vi "Get Display ROI.vi"() -> ()   [LabVIEW 2020]
uses:
  <vilib>/vision/Image Controls.llb/IMAQ Image.ctl
  Documents/Microscope-Control/Display Module/Display Module Custom Controls/ROI Descriptor.ctl
panel:
  out "Y Center":dbl
  out "X Center":dbl
  out "Height":dbl
  out "Width":dbl
  in  "Quit":bool
  out "Error":bool
  in  "Active Image":u16(ring) items=["Channel 101", "Channel 201"]
  out "ROI Data":i32[](array[numeric])
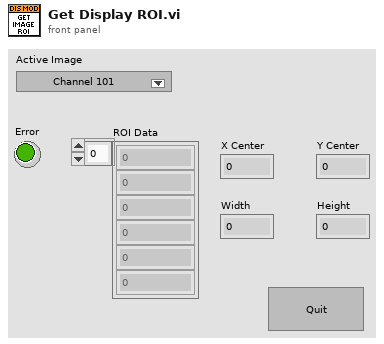
[diagram p1: front panel]
types:
  T1 = typedef "IMAQ Image.ctl" = refnum<image>
  T2 = typedef "ROI Descriptor.ctl" = cluster{"Global Rectangle":i32[], "Contours":cluster{"Contour Type":u32, "ROI Type":u32, "Points":i32[]}[]}
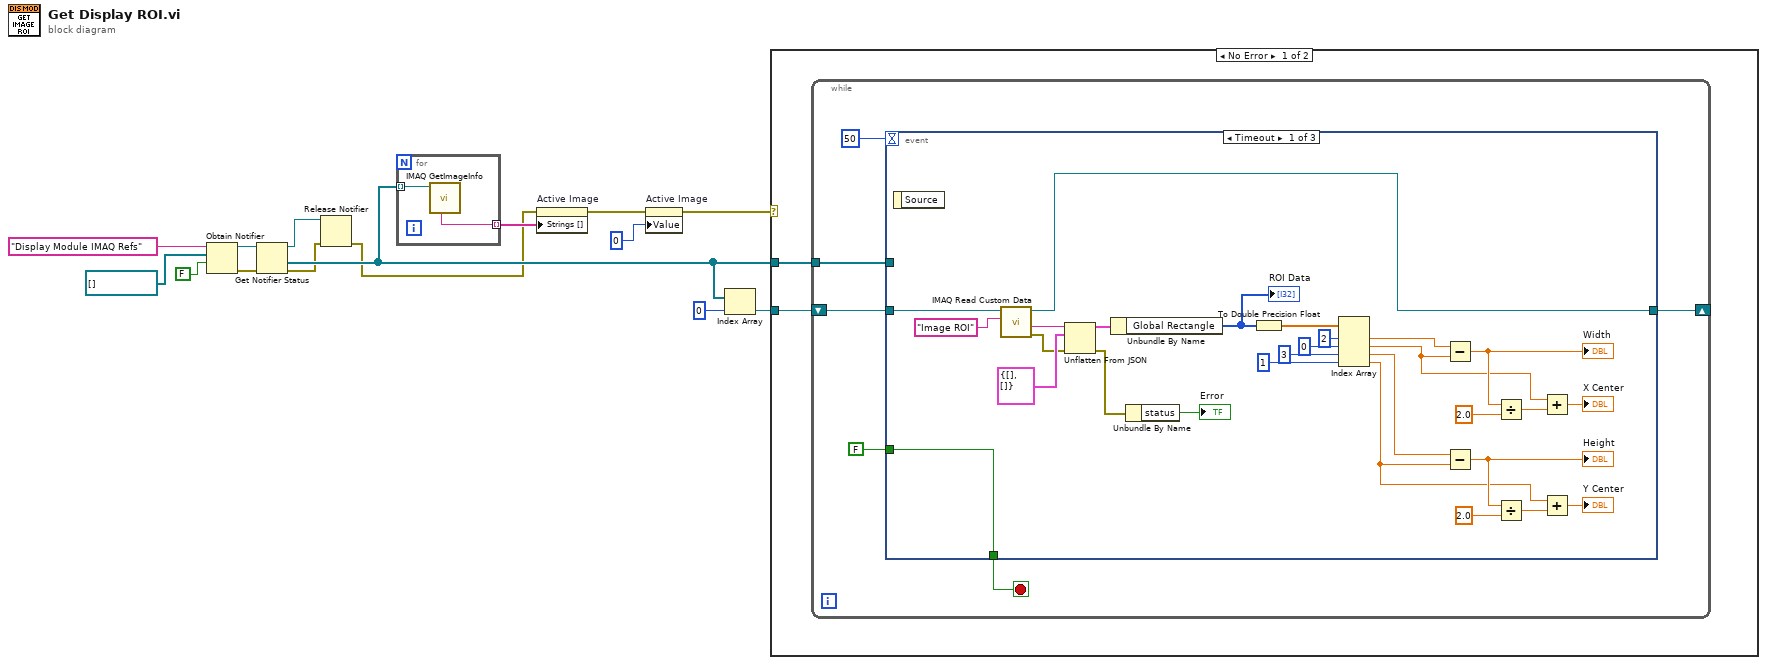
[diagram p0: block diagram]
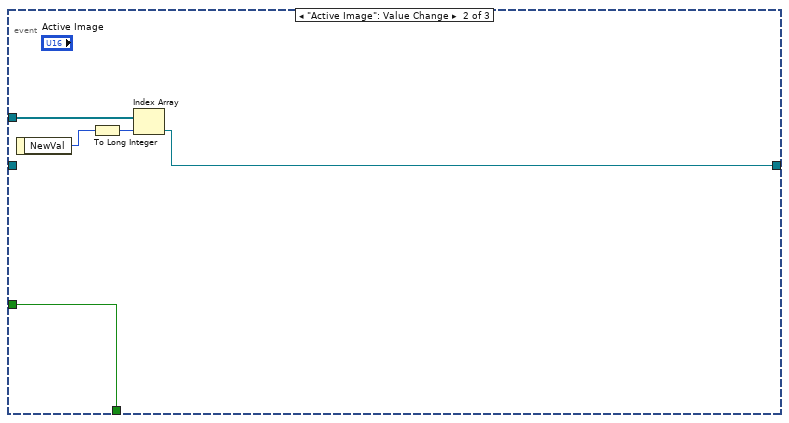
[diagram p2: hidden frame]
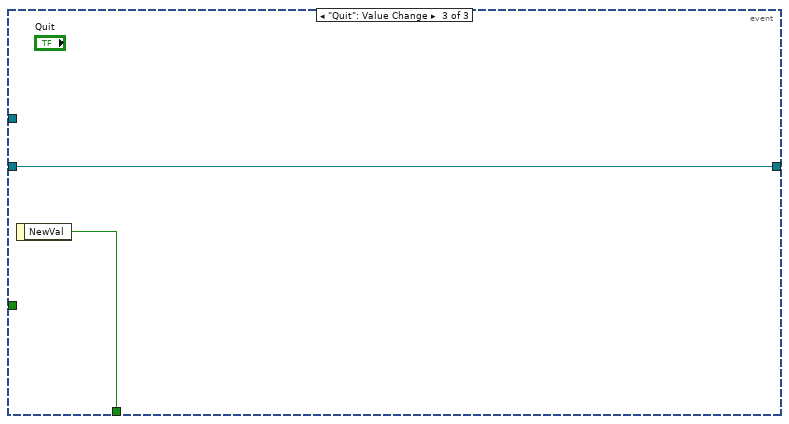
[diagram p3: hidden frame]
diagram:
  n1 = Obtain Notifier(name (unnamed)="Display Module IMAQ Refs", notification data type=T1[] [], create if not found? (T)=FALSE) -> (notifier out=w15:refnum<notifier>, error out=w14:errorcluster)  [unwired: 1 in, 1 out]
  n2 = Get Notifier Status(notifier=w15, error in (no error)=w14) -> (notifier out=w3:refnum<notifier>, current notification=w8:T1[], error out=w2:errorcluster)  [unwired: 2 out]
  n3 = Release Notifier(notifier=w3, error in (no error)=w2) -> (error out=w1:errorcluster)  [unwired: 1 in, 2 out]
  n4 = for {
    tunnel: w8 -> [w17] mode=indexing
    tunnel: [w16] -> w7 mode=indexing
    n5 = call "IMAQ GetImageInfo"("Image"=w17) -> ("Image Name"=w16:string)  [unwired: 3 in, 7 out]
  }
  n6 = property on="Active Image" class="Ring (strict)"(error in=w1, "Strings []"=w7) -> (error out=w5:errorcluster)  [unwired: 1 in, 1 out]
  n7 = property on="Active Image" class="Ring (strict)"(error in=w5, "Value"=u16 0) -> (error out=w4:errorcluster)  [unwired: 1 in, 1 out]
  n8 = Index Array(array=w8, index=0) -> (element=w9:T1)
  n9 = case shown="No Error" w4 {
    tunnel: w9 -> [w19 _]
    tunnel: w8 -> [w18 _]
    frame No Error {
      n10 = while {
        shift-right: [w22] -> _
        shift-left: w19 -> [w23]
        tunnel: w18 -> [w24]
        stop <- w20 stop-if-true
        n11 = event shown="[0] Timeout" {
          selector: _ -> [_ _ _]
          dyn-events: _ -> [_ _ _]
          timeout: 50 -> [_ _ _]
          tunnel: w24 -> [_ w57 _]
          tunnel: w23 -> [w43 _ w59]
          tunnel: [w42 w54 w59] -> w22
          tunnel: FALSE -> [w39 w58 _]
          tunnel: [w39 w58 w60] -> w20
          event Timeout {
            n12 = event-data() -> ()  [unwired: 1 in, 1 out]
            n13 = call "IMAQ Read Custom Data"("Key"="Image ROI", "Image"=w43) -> ("error out"=w44:errorcluster, "Custom Data Out"=w52:string, "Image (duplicate)"=w42:T1)  [unwired: 7 in]
            n14 = Unflatten From JSON(JSON string=w52, type and defaults=T2 {"Global Rectangle"=[], "Contours"=[]} ("Image ROI Descriptor"), error in (no error)=w44) -> (value=w50:T2, error out=w41:errorcluster)  [unwired: 4 in]
            n15 = Unbundle By Name(w50) -> ("Global Rectangle"=w49:i32[])
            "ROI Data" <- w49
            n16 = Unbundle By Name(w41) -> ("status"=→"Error":bool)
            n17 = To Double Precision Float(number=w49) -> (double precision float=w26:dbl[])
            n18 = Index Array(array=w26, index #1=2 ("index"), index #2=0 ("index"), index #3=3 ("index"), index #4=1 ("index")) -> (element #1=w29:dbl, element #2=w30:dbl, element #3=w31:dbl, element #4=w32:dbl)
            n19 = Subtract(x=w29, y=w30) -> (x-y=w38:dbl)
            "Width" <- w38
            n20 = Subtract(x=w31, y=w32) -> (x-y=w35:dbl)
            "Height" <- w35
            n21 = Divide(x=w38, y=2.0) -> (x/y=w28:dbl)
            n22 = Divide(x=w35, y=2.0) -> (x/y=w27:dbl)
            n23 = Add(x=w30, y=w28) -> (x+y=→"X Center":dbl)
            n24 = Add(x=w32, y=w27) -> (x+y=→"Y Center":dbl)
          }
          event "Active Image": Value Change {
            n25 = event-data() -> ("NewVal"=w56:u16)  [unwired: 1 in]
            n26 = To Long Integer(number=w56) -> (32bit integer=w55:i32)
            n27 = Index Array(array=w57, index=w55) -> (element=w54:T1)
          }
          event "Quit": Value Change {
            n28 = event-data() -> ("NewVal"=w60:bool)  [unwired: 1 in]
          }
        }
      }
    }
    frame Error {
    }
  }
